vi "AggregateWaveforms.vi"(6 "new waveforms":waveform(sgl)[](array[waveform]), 8 "samples per block":dbl, 9 "block count":i32, 11 "aggregate waveforms":waveform(sgl)[](array[waveform])) -> (3 "aggregate waveforms out":waveform(sgl)[](array[waveform]))   [LabVIEW 2017, in "CmsAcquisition.lvlib"]
uses:
  <vilib>/addons/InsightCM/Devices/Shared/Cms/CmsAcquisition/CmsAcquisition.lvlib
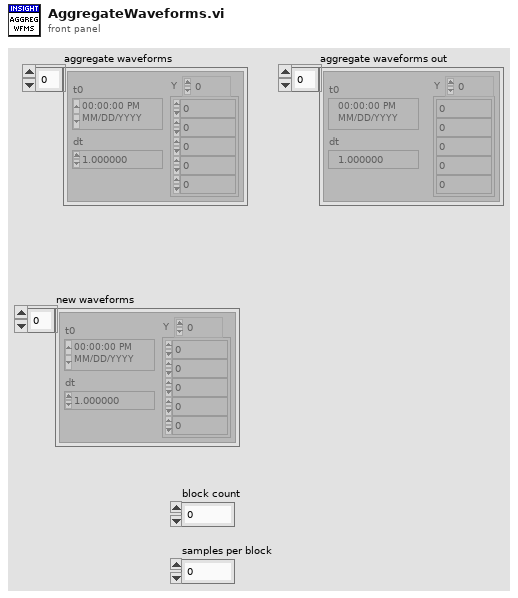
[diagram p1: front panel]
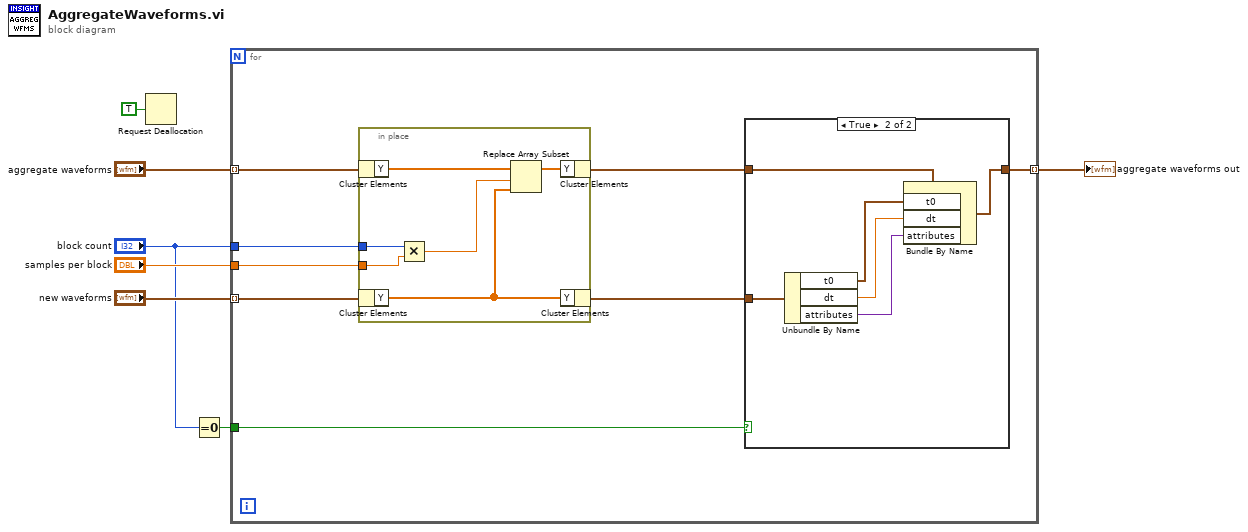
[diagram p0: block diagram]
diagram:
  n1 = Request Deallocation(TRUE ("flag")) -> ()
  n2 = Equal To 0?(x="block count") -> (x = 0?=w3:bool)
  n3 = for {
    tunnel: "aggregate waveforms" -> [w15] mode=indexing
    tunnel: "new waveforms" -> [w14] mode=indexing
    tunnel: "block count" -> [w11]
    tunnel: "samples per block" -> [w13]
    tunnel: [w10] -> w7 mode=indexing
    tunnel: w3 -> [w8]
    n4 = in-place {
      in-place-border: w13 -> [w16]
      in-place-border: w11 -> [w17]
      n5 = in-place-cluster #1(w15) -> ("Y"=w21:sgl[])
      n6 = in-place-cluster #2(w14) -> ("Y"=w18:sgl[])
      n7 = Multiply(x=w17, y=w16) -> (x*y=w20:dbl)
      n8 = Replace Array Subset(array=w21, new element=w18, index=w20) -> (w19:sgl[])
      n9 = in-place-cluster #1("Y"=w19) -> (w12:waveform(sgl))
      n10 = in-place-cluster #2("Y"=w18) -> (w9:waveform(sgl))
    }
    n11 = case shown="True" w8 {
      tunnel: w12 -> [w22 w28]
      tunnel: [w22 w27] -> w10
      tunnel: w9 -> [_ w26]
      frame False {
      }
      frame True {
        n12 = Unbundle By Name(w26) -> ("t0"=w25:timestamp, "dt"=w24:dbl, "attributes"=w23:variant)
        n13 = Bundle By Name(cluster=w28, "t0"=w25, "dt"=w24, "attributes"=w23) -> (w27:waveform(sgl))
      }
    }
  }
  "aggregate waveforms out" <- w7
